vi "Configure HSDIO Gen and Acq w_Script_w Logic Family Input_Selectable SDATA Idle State.vi"(5 "SDATA_Idle_State":enum16{"0", "High Z"}(ring), 7 "logic family":T1=81 items=["5.0V Logic"=5, "3.3V Logic"=6, "2.5V Logic"=7, "1.8V Logic"=8, "1.5V Logic"=80, "1.2V Logic"=81], 8 "error in (no error)":errorcluster, 9 "Clock Rate":dbl=50000000.0 format="%.2p", 10 "Pins":string[](array[string]), 11 "Semiconductor Module Context":T2) -> (0 "error out":errorcluster)   [LabVIEW 2013]
uses:
  <vilib>/NI_TestStand_SemiconductorModule/NI_TestStand_Semiconductor_Module.lvlibp/PinMap/General/SemiconductorModuleContext.ctl
  <instrlib>/niHSDIO/niHSDIO.llb/niHSDIO_ctl Voltage Logic Family Values (Ring).ctl
  <instrlib>/niHSDIO/niHSDIO.llb/niHSDIO_ctl Trigger Script - trigID Values (Ring).ctl
  <instrlib>/niHSDIO/niHSDIO.llb/niHSDIO_ctl Generation Mode Values (Ring).ctl
  <instrlib>/niHSDIO/niHSDIO.llb/niHSDIO_ctl Data Position Values (Ring).ctl
  <instrlib>/niHSDIO/niHSDIO.llb/niHSDIO_ctl Trigger Source Values (Ring).ctl
  <instrlib>/niHSDIO/niHSDIO.llb/niHSDIO_ctl Exported Signal Name Values (Ring).ctl
  <vilib>/NI_TestStand_SemiconductorModule/NI_TestStand_Semiconductor_Module.lvlibp/PinMap/HSDIO/PinsToNIHSDIOSessions.vi
  <instrlib>/niHSDIO/niHSDIO.llb/niHSDIO Configure Digital Edge Start Trigger.vi
  <instrlib>/niHSDIO/niHSDIO.llb/niHSDIO Configure Data Voltage Logic Family.vi
  <instrlib>/niHSDIO/niHSDIO.llb/niHSDIO Configure Software Script Trigger.vi
  <instrlib>/niHSDIO/niHSDIO.llb/niHSDIO Configure Initial State (String).vi
  <instrlib>/niHSDIO/niHSDIO.llb/niHSDIO Configure Idle State (String).vi
  <vilib>/NI_TestStand_SemiconductorModule/NI_TestStand_Semiconductor_Module.lvlibp
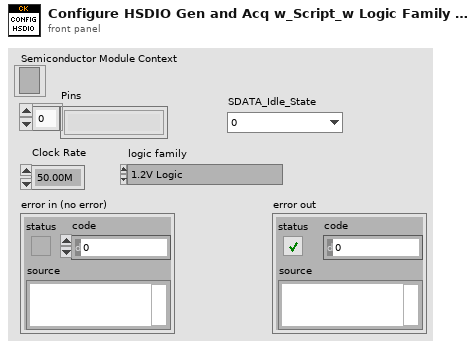
[diagram p1: front panel]
types:
  T1 = typedef "niHSDIO_ctl Voltage Logic Family Values (Ring).ctl" = i32
  T2 = typedef "NI_TestStand_Semiconductor_Module.lvlibp/SemiconductorModuleContext.ctl" = refnum<k7>
  T3 = typedef "niHSDIO_ctl Trigger Script - trigID Values (Ring).ctl" = string
  T4 = typedef "niHSDIO_ctl Exported Signal Name Values (Ring).ctl" = u16
  T5 = typedef "niHSDIO_ctl Trigger Source Values (Ring).ctl" = string
  T6 = typedef "niHSDIO_ctl Data Position Values (Ring).ctl" = i32
  T7 = typedef "niHSDIO_ctl Generation Mode Values (Ring).ctl" = i32
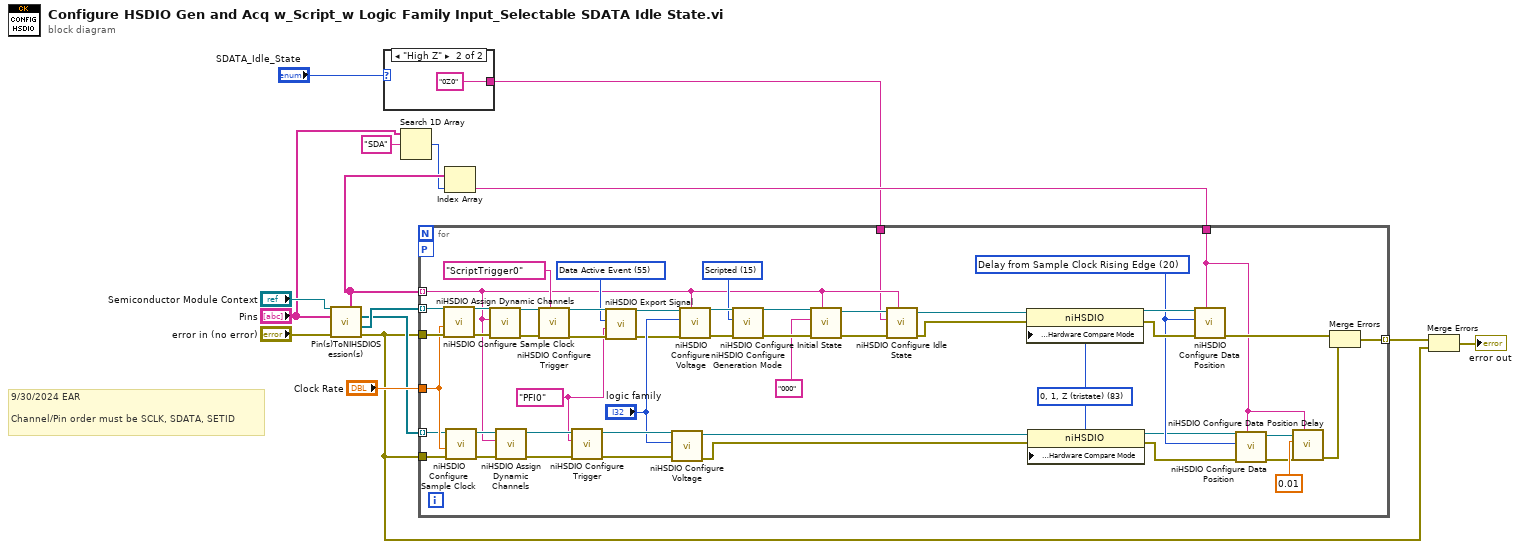
[diagram p0: block diagram]
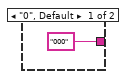
[diagram p2: hidden frame]
diagram:
  # "9/30/2024 EAR\n\nChannel/Pin order must be SCLK, SDATA, SETID"
  n1 = call-poly <vilib>:"Pin(s)ToNIHSDIOSession(s).vi"("error in (no error)"="error in (no error)", "Pins"="Pins", "Semiconductor Module Context"="Semiconductor Module Context") -> ("error out"=w9:errorcluster, "Generation Sessions"=w15:refnum<k15>[], "Acquisition Sessions"=w10:refnum<k15>[], "Channel Lists"=w4:string[])  [unwired: 3 in, 2 out]
  n2 = case shown="\"High Z\"" "SDATA_Idle_State" {
    tunnel: ["000" ("initial state") "0Z0" ("idle state")] -> w1
    frame "0", Default {
    }
    frame "High Z" {
    }
  }
  n3 = Search 1D Array(1D array="Pins", element="SDA") -> (index of element=w3:i32)  [unwired: 1 in]
  n4 = Index Array(array=w4, index=w3) -> (element=w5:string)
  n5 = for {
    tunnel: w4 -> [w19] mode=indexing
    tunnel: w15 -> [w66] mode=indexing
    tunnel: "Clock Rate" -> [w55]
    workers-P: _ -> [_]
    tunnel: w9 -> [w67]
    tunnel: w10 -> [w54] mode=indexing
    tunnel: w9 -> [w53]
    tunnel: [w26] -> w8 mode=indexing
    tunnel: w5 -> [w25]
    tunnel: w1 -> [w18]
    w30 = T4 55 items=["Sample Clock"=51, "Reference Clock"=52, "Start Trigger"=53, "Reference Trigger"=54, "Advance Trigger"=61, "Pause Trigger"=57, "Script Trigger"=58, "Stop Trigger"=82, "Data Active Event"=55, "Marker Event"=59, "Ready For Start Event"=56, "Ready For Advance Event"=66, "End Of Record Event"=68, "Onboard Ref Clock"=60] ("signal (sample clock)")
    w29 = T5 "PFI0" ("source (PFI 0)")
    w43 = 83 items=["0, 1 (binary)"=77, "0, 1, Z (tristate)"=83, "0, 1, Z, L, H, X (stim/resp)"=78, "L, H, X (resp only)"=79] ("Advanced:Supported Data States")
    w39 = T6 20 items=["Sample Clock Rising Edge"=18, "Sample Clock Falling Edge"=19, "Delay from Sample Clock Rising Edge"=20] ("position (rising edge)")
    w58 = T7 15 items=["Waveform"=14, "Scripted"=15] ("generation mode (waveform)")
    n6 = call <instrlib>:"niHSDIO Configure Sample Clock.vi"("error in (no error)"=w67, "clock rate (50MHz)"=w55, "instrument handle"=w66) -> ("error out"=w65:errorcluster, "instrument handle out"=w64:refnum<k15>)  [unwired: 7 in]
    n7 = call <instrlib>:"niHSDIO Configure Sample Clock.vi"("error in (no error)"=w53, "clock rate (50MHz)"=w55, "instrument handle"=w54) -> ("error out"=w52:errorcluster, "instrument handle out"=w51:refnum<k15>)  [unwired: 7 in]
    n8 = call <instrlib>:"niHSDIO Assign Dynamic Channels.vi"("error in (no error)"=w65, "channel list (all:\"\")"=w19, "instrument handle"=w64) -> ("error out"=w63:errorcluster, "instrument handle out"=w62:refnum<k15>)  [unwired: 7 in]
    n9 = call <instrlib>:"niHSDIO Assign Dynamic Channels.vi"("error in (no error)"=w52, "channel list (all:\"\")"=w19, "instrument handle"=w51) -> ("error out"=w49:errorcluster, "instrument handle out"=w50:refnum<k15>)  [unwired: 7 in]
    n10 = call-poly <instrlib>:"niHSDIO Configure Trigger.vi"("trigger id (script trigger 0)"=T3 "ScriptTrigger0", "error in (no error)"=w63, "instrument handle"=w62) -> ("error out"=w31:errorcluster, "instrument handle out"=w34:refnum<k15>)  [unwired: 7 in]
    n11 = call-poly <instrlib>:"niHSDIO Configure Trigger.vi"("error in (no error)"=w49, "source (PFI 0)"=w29, "instrument handle"=w50) -> ("error out"=w48:errorcluster, "instrument handle out"=w47:refnum<k15>)  [unwired: 7 in]
    n12 = call <instrlib>:"niHSDIO Export Signal.vi"("error in (no error)"=w31, "output terminal (do not export)"=w29, "signal (sample clock)"=w30, "instrument handle"=w34) -> ("error out"=w32:errorcluster, "instrument handle out"=w33:refnum<k15>)  [unwired: 6 in]
    n13 = call-poly <instrlib>:"niHSDIO Configure Voltage.vi"("error in (no error)"=w48, "logic family (3.3V logic)"="logic family", "instrument handle"=w47) -> ("error out"=w41:errorcluster, "instrument handle out"=w42:refnum<k15>)  [unwired: 7 in]
    n14 = call-poly <instrlib>:"niHSDIO Configure Voltage.vi"("channel list (all:\"\")"=w19, "error in (no error)"=w32, "logic family (3.3V logic)"="logic family", "instrument handle"=w33) -> ("error out"=w60:errorcluster, "instrument handle out"=w59:refnum<k15>)  [unwired: 6 in]
    n15 = call <instrlib>:"niHSDIO Configure Generation Mode.vi"("error in (no error)"=w60, "generation mode (waveform)"=w58, "instrument handle"=w59) -> ("error out"=w57:errorcluster, "instrument handle out"=w56:refnum<k15>)  [unwired: 7 in]
    n16 = call-poly <instrlib>:"niHSDIO Configure Initial State.vi"("channel list"=w19, "error in (no error)"=w57, "initial state"="000", "instrument handle"=w56) -> ("error out"=w24:errorcluster, "instrument handle out"=w23:refnum<k15>)  [unwired: 6 in]
    n17 = call-poly <instrlib>:"niHSDIO Configure Idle State.vi"("channel list"=w19, "error in (no error)"=w24, "idle state"=w18, "instrument handle"=w23) -> ("error out"=w21:errorcluster, "instrument handle out"=w20:refnum<k15>)  [unwired: 6 in]
    n18 = property on="Property Node" class="niHSDIO"(reference=w20, error in=w21, "Advanced:Hardware Compare:Hardware Compare Mode"=w43) -> (reference out=w45:refnum<k15>, error out=w44:errorcluster)
    n19 = property on="Property Node" class="niHSDIO"(reference=w42, error in=w41, "Advanced:Hardware Compare:Hardware Compare Mode"=w43) -> (reference out=w36:refnum<k15>, error out=w40:errorcluster)
    n20 = call <instrlib>:"niHSDIO Configure Data Position.vi"("channel list (all:\"\")"=w25, "error in (no error)"=w44, "position (rising edge)"=w39, "instrument handle"=w45) -> ("error out"=w28:errorcluster)  [unwired: 6 in, 1 out]
    n21 = call <instrlib>:"niHSDIO Configure Data Position.vi"("channel list (all:\"\")"=w25, "error in (no error)"=w40, "position (rising edge)"=w39, "instrument handle"=w36) -> ("error out"=w35:errorcluster, "instrument handle out"=w37:refnum<k15>)  [unwired: 6 in]
    n22 = call <instrlib>:"niHSDIO Configure Data Position Delay.vi"("channel list (all:\"\")"=w25, "error in (no error)"=w35, "delay (0.000)"=0.01, "instrument handle"=w37) -> ("error out"=w27:errorcluster)  [unwired: 6 in, 1 out]
    n23 = Merge Errors(w28, w27) -> (w26:errorcluster)
  }
  n24 = Merge Errors(w8, w9) -> (→"error out":errorcluster)
